vi "Set_Parameter_Instrument (Json).vi"(8 "error in (no error)":errorcluster caption="entrée d'erreur (pas d'erreur)", 10 "Parameter (Json)":string, 11 "Start Blink_Relay en entrée":refnum<class "Start_Blink_Relay.lvclass">) -> (0 "error out":errorcluster caption="sortie d'erreur", 3 "Start Blink_Relay en sortie":refnum<class "Start_Blink_Relay.lvclass">)   [LabVIEW 2020, in "Library Test.lvlib" / "Start_Blink_Relay.lvclass"]
uses:
  Start_Blink_Relay.lvclass
  C:/Users/ngarcin/OneDrive - Altyor/Standard TB/Class/Test/Test (Default)/Test (Default).lvclass
  Commun VI/TypeDef/Commande Relay_Board/Parameter Relay_Board.ctl
  Relay_Board/Relay_Board (Default)/Class Relay_Board (Default).lvclass
  Start_Blink_Relay.lvclass/Start_Blink_Relay.ctl
  JSON API/JSON Value/Set from JSON string.vi
  JSON API/Variant JSON/Variant to JSON.vi
  JSON API/JSON Value/Get Item by name array.vi
  Test_Wtih_Instr/Test_With_Inst.lvclass
  Instrument/Instrument (Default)/Class Instrument (Default).lvclass
  JSON API/JSON Value/JSON Value.lvclass
  JSON API/Variant JSON/Variant JSON.lvlib
  JSON API/Get Polymorphic/JSON GetSet.lvlib
  Commun VI/Library Commun.lvlib
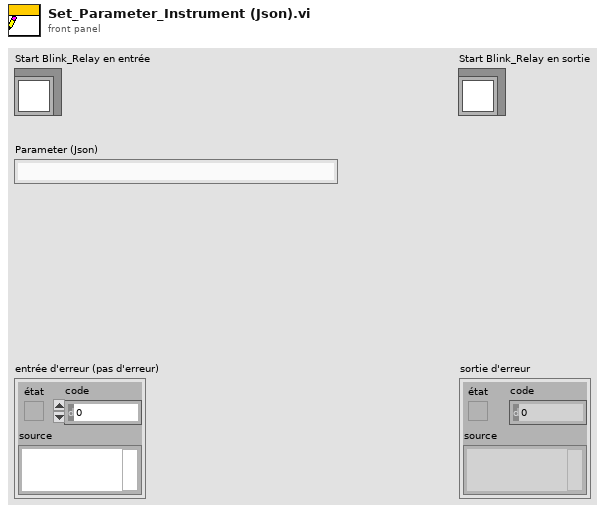
[diagram p1: front panel]
types:
  T1 = typedef "Library Commun.lvlib/Parameter Relay_Board.ctl" = cluster{"Device_Com_Port":string, "Address Board":string, "Tab_Num_Relay":u8[], "Parameter Class Relay_Board":refnum<class "Class Relay_Board (Default).lvclass">}
  T2 = cluster{"Time On":u16, "Time Off":u16, "Relay":i32}
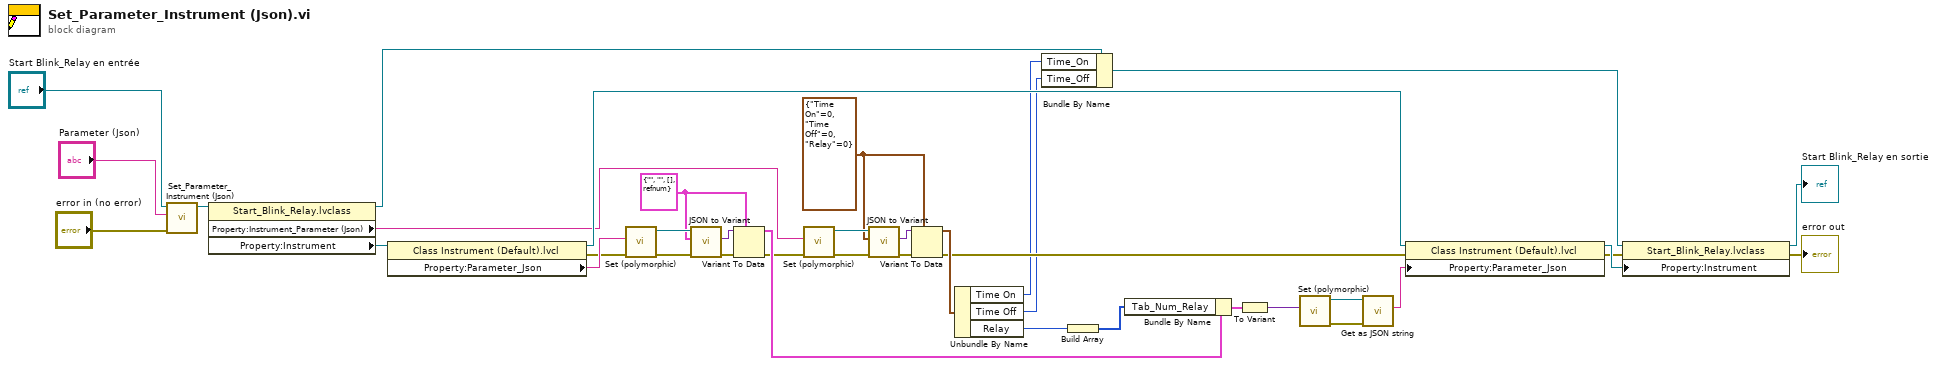
[diagram p0: block diagram]
diagram:
  w21 = T1 {"Device_Com_Port"="", "Address Board"="", "Tab_Num_Relay"=[], "Parameter Class Relay_Board"=refnum} ("Parameter")
  w30 = T2 {"Time On"=0, "Time Off"=0, "Relay"=0} ("Cluster des données privées de classe")
  n1 = call-parent "Set_Parameter_Instrument (Json).vi"("error in (no error)"="error in (no error)", "Parameter (Json)"="Parameter (Json)", "Test (Default) en entrée"="Start Blink_Relay en entrée") -> ("Test (Default) en sortie"=w35:refnum<class "Start_Blink_Relay.lvclass">)  [unwired: 7 in, 1 out]
  n2 = property class="Start_Blink_Relay.lvclass"(reference=w35) -> (reference out=w5:refnum<class "Start_Blink_Relay.lvclass">, "Property:Instrument_Parameter (Json)"=w14:string, "Property:Instrument"=w15:refnum<class "Class Instrument (Default).lvclass">)  [unwired: 1 in, 1 out]
  n3 = property class="Class Instrument (Default).lvcl"(reference=w15) -> (reference out=w29:refnum<class "Class Instrument (Default).lvclass">, error out=w23:errorcluster, "Property:Parameter_Json"=w24:string)  [unwired: 1 in]
  n4 = call-poly "Set (polymorphic).vi"("error in (no error)"=w23, "JSON stream"=w24) -> ("error out"=w26:errorcluster, "JSON Value out"=w28:refnum<class "JSON Value.lvclass">)  [unwired: 7 in, 1 out]
  n5 = call "JSON to Variant.vi"("error in (no error)"=w26, "Variant (Data Type)"=w21, "JSON Value"=w28) -> ("error out"=w27:errorcluster, "Variant out"=w25:variant)  [unwired: 7 in]
  n6 = Variant To Data(error in=w27, type=w21, Variant=w25) -> (data=w22:T1, error out=w11:errorcluster)
  n7 = call-poly "Set (polymorphic).vi"("error in (no error)"=w11, "JSON stream"=w14) -> ("error out"=w33:errorcluster, "JSON Value out"=w31:refnum<class "JSON Value.lvclass">)  [unwired: 7 in, 1 out]
  n8 = call "JSON to Variant.vi"("error in (no error)"=w33, "Variant (Data Type)"=w30, "JSON Value"=w31) -> ("error out"=w32:errorcluster, "Variant out"=w34:variant)  [unwired: 7 in]
  n9 = Variant To Data(error in=w32, type=w30, Variant=w34) -> (data=w13:T2, error out=w10:errorcluster)
  n10 = Unbundle By Name(w13) -> ("Time On"=w3:u16, "Time Off"=w2:u16, "Relay"=w12:i32)
  n11 = Bundle By Name(cluster=w5, "Time_On"=w3, "Time_Off"=w2) -> (w4:refnum<class "Start_Blink_Relay.lvclass">)
  n12 = Build Array(w12) -> (w20:i32[])
  n13 = Bundle By Name(cluster=w22, "Tab_Num_Relay"=w20) -> (w18:T1)
  n14 = To Variant(anything=w18) -> (Variant=w17:variant)
  n15 = call-poly "Set (polymorphic).vi"("Variant"=w17) -> ("error out"=w1:errorcluster, "JSON Value out"=w19:refnum<class "JSON Value.lvclass">)  [unwired: 9 in]
  n16 = call "Get as JSON string.vi"("error in (no error)"=w1, "JSON Value in"=w19) -> ("<JSON>"=w16:string)  [unwired: 8 in, 1 out]
  n17 = property class="Class Instrument (Default).lvcl"(reference=w29, error in=w10, "Property:Parameter_Json"=w16) -> (reference out=w9:refnum<class "Class Instrument (Default).lvclass">, error out=w8:errorcluster)
  n18 = property class="Start_Blink_Relay.lvclass"(reference=w4, error in=w8, "Property:Instrument"=w9) -> (reference out=→"Start Blink_Relay en sortie":refnum<class "Start_Blink_Relay.lvclass">, error out=→"error out":errorcluster)
